vi "testlooslescomp.vi"() -> ()   [LabVIEW 2009]
uses:
  <vilib>/vision/Image Controls.llb/IMAQ Image.ctl
panel:
  out "tosend 3":T1(plugin-control)
  in  "Compression (None)":i32(ring) items=["None", "JPEG", "PACKED BINARY"]
  in  "Type of Flatten (Image and Vision Info)":i32(ring)=1 items=["Image", "Image and Vision Info", "Reference to Image"]
  out "Data String":string
  in  "tosend 2":T1(plugin-control)
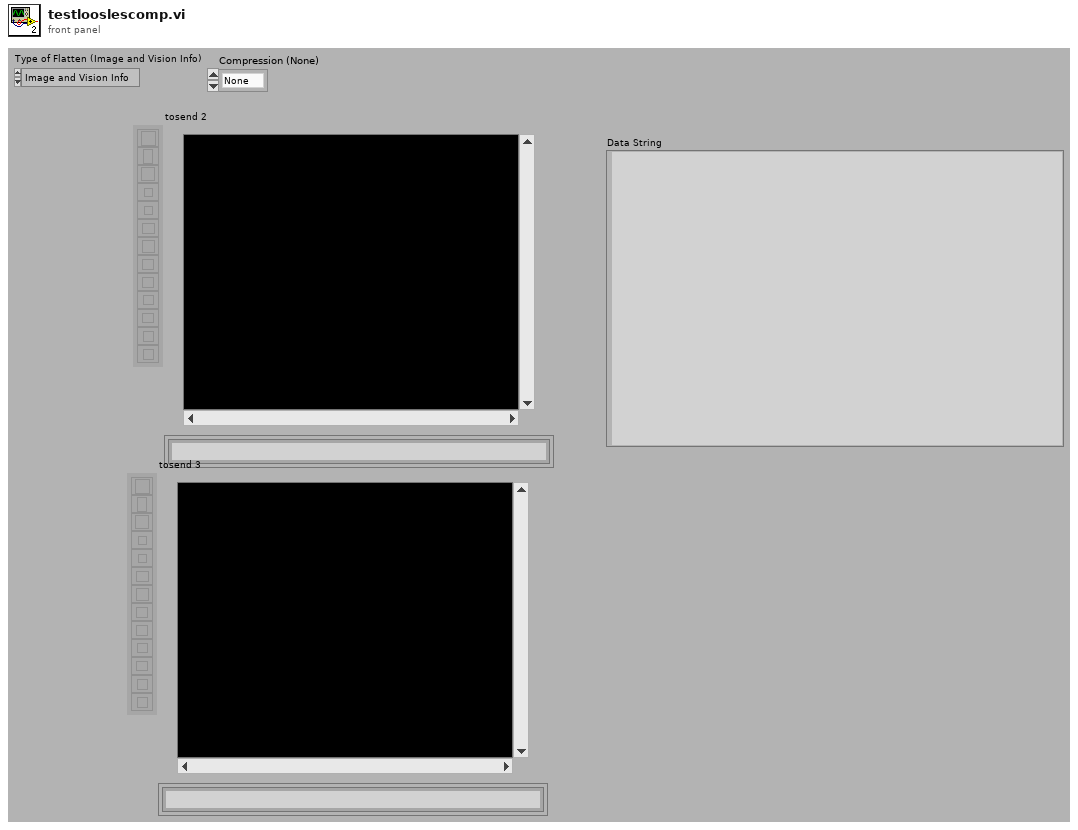
[diagram p1: front panel]
types:
  T1 = typedef "IMAQ Image.ctl" = refnum<image>
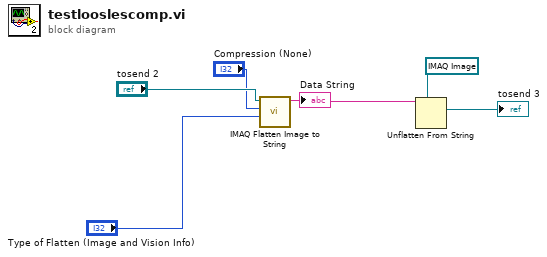
[diagram p0: block diagram]
diagram:
  n1 = call "IMAQ Flatten Image to String"("Type of Flatten (Image and Vision Info)"="Type of Flatten (Image and Vision Info)", "Compression (None)"="Compression (None)", "Image"="tosend 2") -> ("Data String"=w3:string)  [unwired: 7 in, 1 out]
  "Data String" <- w3
  n2 = Unflatten From String(type=T1 refnum ("tosend 2"), binary string=w3) -> (value=→"tosend 3":T1)  [unwired: 3 in, 2 out]
